vi "SteeringFrame.vi"() -> (3 "NI_Robotics_Steering Frame out":refnum<class "NI_Robotics_Steering Frame.lvclass">)   [LabVIEW 2018]
uses:
  <vilib>/robotics/Steering/Steering Frame/NI_Robotics_Steering Frame.lvclass
  <vilib>/robotics/Steering/Wheel/Rotation Direction.ctl
  <vilib>/robotics/Steering/Wheel/Wheel Parameters.ctl
  <vilib>/robotics/Steering/Omnidirectional Wheel/NI_Robotics_Omnidirectional Wheel.lvclass
  C:/Program Files (x86)/National Instruments/LabVIEW 2018/vi.lib/robotics/Steering/Wheel/NI_Robotics_Wheel.lvclass
  <vilib>/robotics/Steering/Omnidirectional Wheel/Create Omnidirectional Wheel.vi
  <vilib>/robotics/Steering/Steering Frame/Create User Defined Steering Frame.vi
  <vilib>/robotics/Steering/Wheel/NI_Robotics_Wheel.lvclass
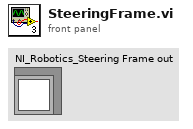
[diagram p1: front panel]
types:
  T1 = typedef "NI_Robotics_Wheel.lvclass/Wheel Parameters.ctl" = cluster{"wheel radius":dbl, "gear ratio":dbl, "forward rotation direction":T2}
  T2 = typedef "NI_Robotics_Wheel.lvclass/Rotation Direction.ctl" = u16
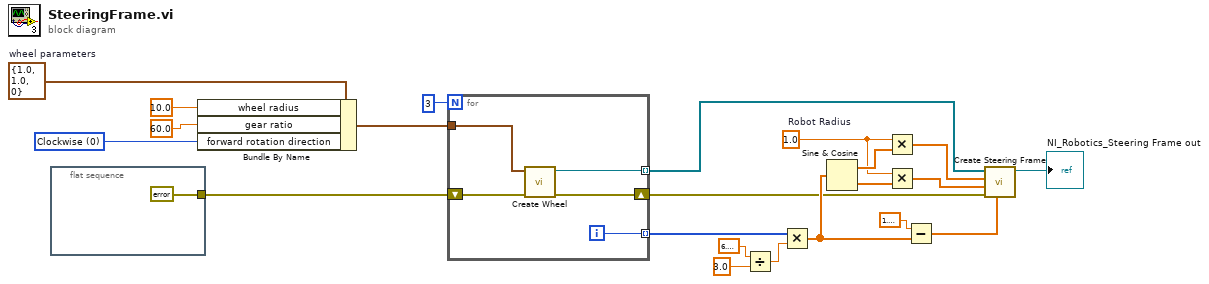
[diagram p0: block diagram]
diagram:
  w1 = T1 {"wheel radius"=1.0, "gear ratio"=1.0, "forward rotation direction"=0}  # wheel parameters
  w16 = T2 0 items=["Clockwise", "Counterclockwise"] ("forward rotation direction")
  w11 = 1.0  # Robot Radius
  n1 = flat-sequence {
    tunnel: [errorcluster {"status"=FALSE, "code"=0, "source"=""} ("error out")] -> w5
    frame #0 {
    }
  }
  n2 = Bundle By Name(cluster=w1, "wheel radius"=10.0, "gear ratio"=60.0, "forward rotation direction"=w16) -> (w4:T1)
  n3 = for {
    N: 3 -> [_]
    shift-right: [w27] -> w18
    shift-left: w5 -> [w28]
    tunnel: [w26] -> w6 mode=indexing
    tunnel: w4 -> [w25]
    tunnel: [w24] -> w10 mode=indexing
    i -> [w24]
    n4 = call-poly <vilib>:"Create Wheel.vi"("error in (no error)"=w28, "wheel parameters"=w25) -> ("error out"=w27:errorcluster, "omni wheel out"=w26:refnum<class "NI_Robotics_Omnidirectional Wheel.lvclass">)  [unwired: 8 in]
  }
  n5 = Divide(x=6.283185307179586, y=3.0) -> (x/y=w9:dbl)
  n6 = Multiply(x=w10, y=w9) -> (x*y=w21:dbl[])
  n7 = Sine & Cosine(0:w21) -> (1:w19:dbl[], 2:w20:dbl[])
  n8 = Multiply(x=w11, y=w19) -> (x*y=w12:dbl[])
  n9 = Multiply(x=w11, y=w20) -> (x*y=w13:dbl[])
  n10 = Subtract(x=1.5707963267948966, y=w21) -> (x-y=w15:dbl[])
  n11 = call-poly <vilib>:"Create Steering Frame.vi"("wheel frame angles (rad)"=w15, "error in (no error)"=w18, "wheel y positions"=w13, "wheel x positions"=w12, "wheels"=w6) -> ("steering frame out"=→"NI_Robotics_Steering Frame out":refnum<class "NI_Robotics_Steering Frame.lvclass">)  [unwired: 5 in, 1 out]
